vi "Create_VI_Documentation_Component_MultiImages.vi"(6 "special chars in file path of image":string, 7 "Content Options":T1, 8 "error in (no error)":errorcluster, 9 "Image Depth":i32=24, 10 "Image Format (jpeg)":enum32{"PNG", "JPEG", "GIF"}(ring)=enum."JPEG", 11 "VI":refnum<vi>) -> (0 "error out":errorcluster, 3 "Paths to images":path[](array[path]))   [LabVIEW 2017, in "NI_ReportGenerationCore.lvlib"]
uses:
  <vilib>/Utility/NIReport.llb/NI_ReportGenerationCore.lvlib
  <vilib>/printing/ReportDocExtensions.llb/File_types_for_reports.ctl
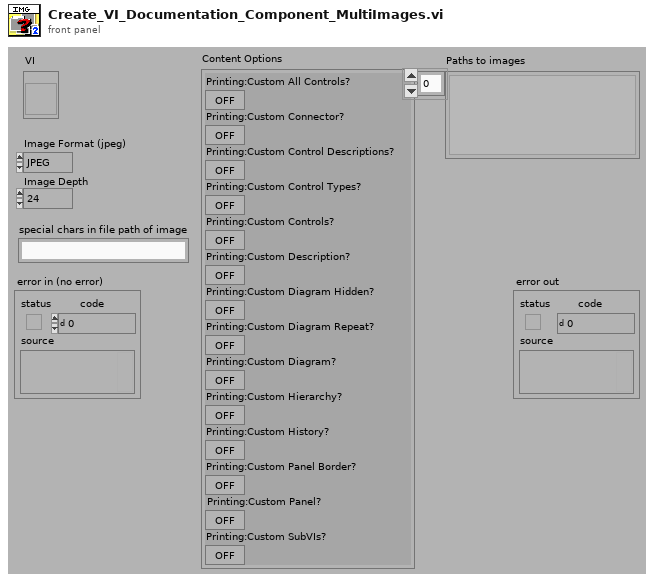
[diagram p1: front panel]
types:
  T1 = cluster{"Printing:Custom All Controls?":bool, "Printing:Custom Connector?":bool, "Printing:Custom Control Descriptions?":bool, "Printing:Custom Control Types?":bool, "Printing:Custom Controls?":bool, "Printing:Custom Description?":bool, "Printing:Custom Diagram Hidden?":bool, "Printing:Custom Diagram Repeat?":bool, "Printing:Custom Diagram?":bool, "Printing:Custom Hierarchy?":bool, "Printing:Custom History?":bool, "Printing:Custom Panel Border?":bool, "Printing:Custom Panel?":bool, "Printing:Custom SubVIs?":bool}
  T2 = typedef "NI_ReportGenerationCore.lvlib/File_types_for_reports.ctl" = enum16{".jpg", ".png", ".html", ".gif"}
  T3 = enum32{"Custom", "Standard", "Using Panel", "Using SubVI", "Complete"}
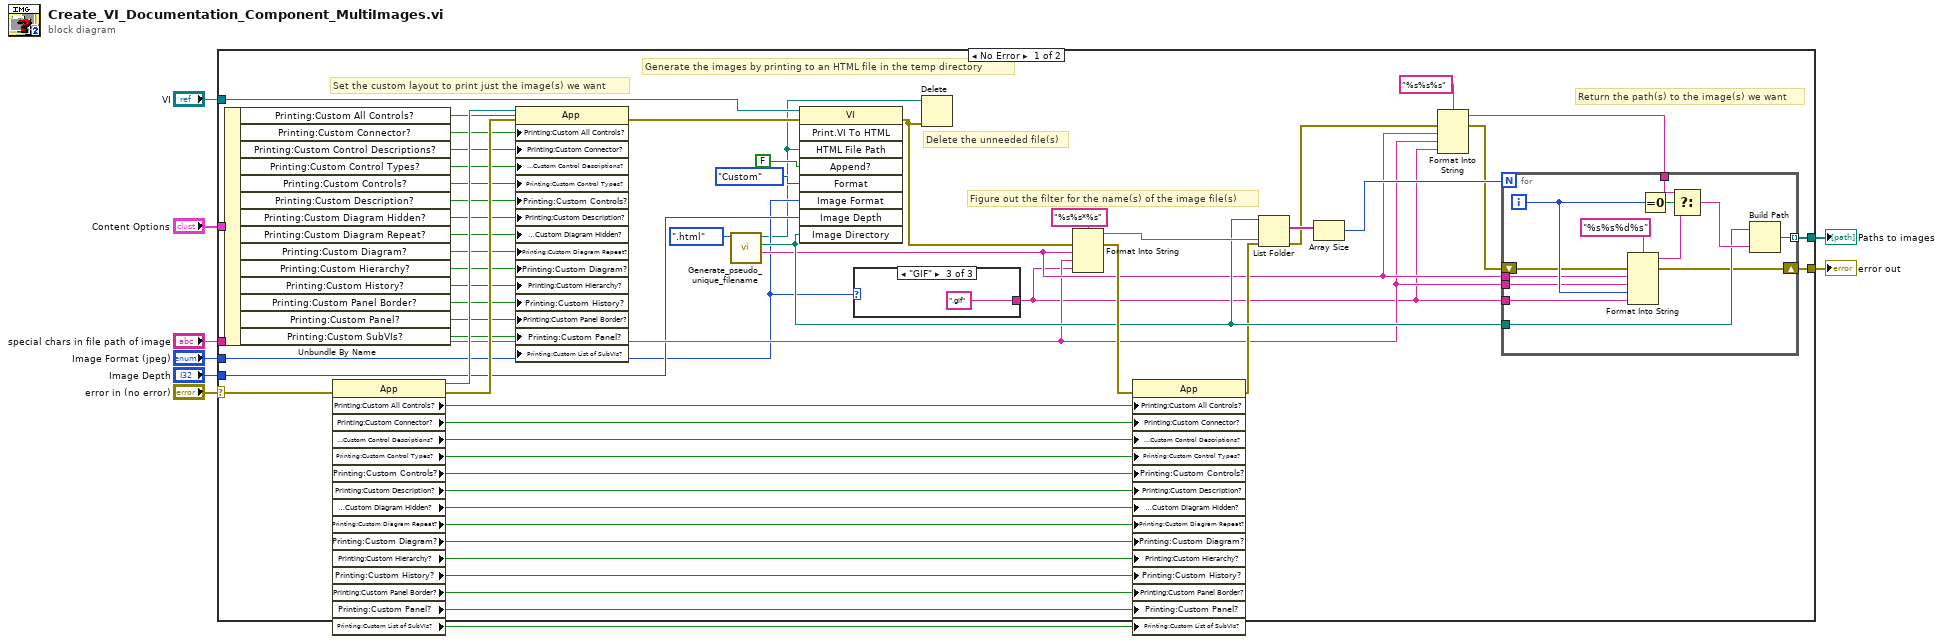
[diagram p0: block diagram]
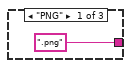
[diagram p2: hidden frame]
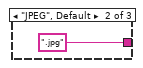
[diagram p3: hidden frame]
diagram:
  n1 = case shown="No Error" "error in (no error)" {
    selector: "error in (no error)" -> [w12 w82]
    tunnel: "VI" -> [w48 _]
    tunnel: "Content Options" -> [w41 _]
    tunnel: "special chars in file path of image" -> [w19 _]
    tunnel: [w16 _] -> w5
    tunnel: [w13 w82] -> w4
    tunnel: "Image Depth" -> [w11 _]
    tunnel: "Image Format (jpeg)" -> [w10 _]
    frame No Error {
      # "Figure out the filter for the name(s) of the image file(s)"
      # "Return the path(s) to the image(s) we want"
      # "Delete the unneeded file(s)"
      # "Generate the images by printing to an HTML file in the temp directory"
      # "Set the custom layout to print just the image(s) we want"
      n2 = Unbundle By Name(w41) -> ("Printing:Custom All Controls?"=w40:bool, "Printing:Custom Connector?"=w39:bool, "Printing:Custom Control Descriptions?"=w38:bool, "Printing:Custom Control Types?"=w37:bool, "Printing:Custom Controls?"=w36:bool, "Printing:Custom Description?"=w35:bool, "Printing:Custom Diagram Hidden?"=w34:bool, "Printing:Custom Diagram Repeat?"=w33:bool, "Printing:Custom Diagram?"=w32:bool, "Printing:Custom Hierarchy?"=w31:bool, "Printing:Custom History?"=w30:bool, "Printing:Custom Panel Border?"=w29:bool, "Printing:Custom Panel?"=w28:bool, "Printing:Custom SubVIs?"=w27:bool)
      n3 = property class="App"(error in=w12) -> (reference out=w51:refnum<vi>, error out=w50:errorcluster, "Printing:Custom All Controls?"=w52:bool, "Printing:Custom Connector?"=w53:bool, "Printing:Custom Control Descriptions?"=w54:bool, "Printing:Custom Control Types?"=w55:bool, "Printing:Custom Controls?"=w56:bool, "Printing:Custom Description?"=w57:bool, "Printing:Custom Diagram Hidden?"=w58:bool, "Printing:Custom Diagram Repeat?"=w59:bool, "Printing:Custom Diagram?"=w60:bool, "Printing:Custom Hierarchy?"=w61:bool, "Printing:Custom History?"=w62:bool, "Printing:Custom Panel Border?"=w63:bool, "Printing:Custom Panel?"=w64:bool, "Printing:Custom List of SubVIs?"=w65:bool)  [unwired: 1 in]
      n4 = property class="App"(reference=w51, error in=w50, "Printing:Custom All Controls?"=w40, "Printing:Custom Connector?"=w39, "Printing:Custom Control Descriptions?"=w38, "Printing:Custom Control Types?"=w37, "Printing:Custom Controls?"=w36, "Printing:Custom Description?"=w35, "Printing:Custom Diagram Hidden?"=w34, "Printing:Custom Diagram Repeat?"=w33, "Printing:Custom Diagram?"=w32, "Printing:Custom Hierarchy?"=w31, "Printing:Custom History?"=w30, "Printing:Custom Panel Border?"=w29, "Printing:Custom Panel?"=w28, "Printing:Custom List of SubVIs?"=w27) -> (error out=w49:errorcluster)  [unwired: 1 out]
      n5 = call <vilib>:"Generate_pseudo_unique_filename.vi"("file type(.jpg)"=File_types_for_reports.".html") -> ("root filename"=w20:string, "temp directory"=w23:path, "generated path"=w9:path)  [unwired: 8 in]
      n6 = invoke class="VI" method="Print.VI To HTML"(reference=w48, error in=w49, "HTML File Path"=w9, "Append?"=FALSE, "Format"=T3."Custom", "Image Format"=w10, "Image Depth"=w11, "Image Directory"=w23) -> (error out=w42:errorcluster)  [unwired: 1 in, 8 out]
      n7 = case shown="\"GIF\"" w10 {
        tunnel: [".png" ".jpg" ".gif"] -> w18
        frame "PNG" {
        }
        frame "JPEG", Default {
        }
        frame "GIF" {
        }
      }
      n8 = Delete(path (use dialog)=w9, error in=w42) -> ()  [unwired: 3 in, 3 out]
      n9 = Format Into String(format string="%s%s*%s" ("Format String"), error in=w42, w20, w19, w18) -> (resulting string=w26:string, error out=w43:errorcluster)  [unwired: 1 in]
      n10 = property class="App"(error in=w43, "Printing:Custom All Controls?"=w52, "Printing:Custom Connector?"=w53, "Printing:Custom Control Descriptions?"=w54, "Printing:Custom Control Types?"=w55, "Printing:Custom Controls?"=w56, "Printing:Custom Description?"=w57, "Printing:Custom Diagram Hidden?"=w58, "Printing:Custom Diagram Repeat?"=w59, "Printing:Custom Diagram?"=w60, "Printing:Custom Hierarchy?"=w61, "Printing:Custom History?"=w62, "Printing:Custom Panel Border?"=w63, "Printing:Custom Panel?"=w64, "Printing:Custom List of SubVIs?"=w65) -> (error out=w22:errorcluster)  [unwired: 1 in, 1 out]
      n11 = List Folder(path=w23, pattern=w26, error in=w22) -> (filenames=w25:string[], error out=w15:errorcluster)  [unwired: 1 in, 2 out]
      n12 = Array Size(array=w25) -> (size(s)=w24:i32)
      n13 = Format Into String(format string="%s%s%s", error in=w15, w20, w19, w18) -> (resulting string=w17:string, error out=w14:errorcluster)  [unwired: 1 in]
      n14 = for {
        N: w24 -> [_]
        tunnel: w23 -> [w69]
        tunnel: w20 -> [w72]
        tunnel: w19 -> [w73]
        tunnel: w18 -> [w74]
        tunnel: w17 -> [w71]
        tunnel: [w68] -> w16 mode=indexing
        shift-right: [w66] -> w13
        shift-left: w14 -> [w67]
        i -> [w76]
        n15 = Format Into String(format string="%s%s%d%s", error in=w67, w72, w73, w76, w74) -> (resulting string=w75:string, error out=w66:errorcluster)  [unwired: 1 in]
        n16 = Equal To 0?(x=w76) -> (x = 0?=w77:bool)
        n17 = Select(t=w71, s=w77, f=w75) -> (s? t:f=w70:string)
        n18 = Build Path(base path=w69, name or relative path=w70) -> (appended path=w68:path)
      }
    }
    frame Error {
    }
  }
  "error out" <- w4
  "Paths to images" <- w5
